vi "Get Beta.vi"(11 "R12":dbl) -> (3 "Beta":dbl)   [LabVIEW 2022 SP3]
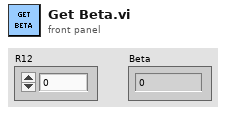
[diagram p1: front panel]
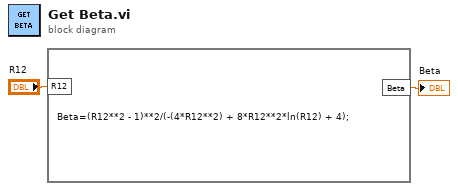
[diagram p0: block diagram]
diagram:
  n1 = formula code="Beta=(R12**2 - 1)**2/(-(4*R12**2) + 8*R12**2*ln(R12) + 4);"("R12"="R12") -> ("Beta"=→"Beta":dbl)
